vi "sync init shared memory.vi"(7 "permissions (0664)":T1={"owner"={"read"=TRUE, "write"=TRUE, "execute"=FALSE}, "group"={"read"=TRUE, "write"=TRUE, "execute"=FALSE}, "everyone"={"read"=TRUE, "write"=TRUE, "execute"=FALSE}}, 8 "error in (no error)":errorcluster, 11 "sync shm name":string) -> (0 "error out":errorcluster, 2 "pointer to shared memory":u64, 3 "shared memory out":T3)   [LabVIEW 2014, in "Shared Memory runtime.lvclass"]
uses:
  Shared Memory runtime.lvclass
  <vilib>/NI/NI Linux RT IPC/Shared Memory/Classes/Shared Memory/Public/Controls/reference.ctl
  <vilib>/NI/NI Linux RT IPC/Shared Memory/Classes/Shared Memory/Shared Memory.lvclass
  <vilib>/NI/NI Linux RT IPC/Shared Memory/Classes/Shared Memory/Public/Controls/permissions group.ctl
  <vilib>/NI/NI Linux RT IPC/Shared Memory/Classes/Shared Memory/Public/Controls/permissions.ctl
  <vilib>/NI/NI Linux RT IPC/Shared Memory/Classes/Shared Memory/Public/Controls/file mode.ctl
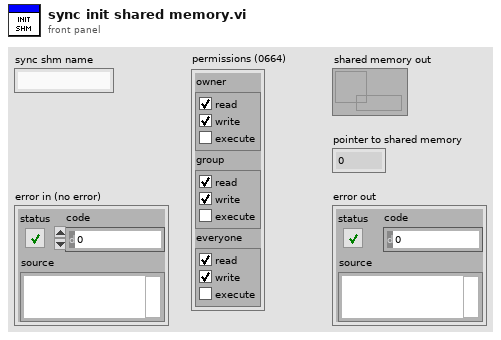
[diagram p1: front panel]
types:
  T1 = typedef "Shared Memory.lvlib/Shared Memory.lvclass/permissions group.ctl" = cluster{"owner":T2, "group":T2, "everyone":T2}
  T2 = typedef "Shared Memory.lvlib/Shared Memory.lvclass/permissions.ctl" = cluster{"read":bool, "write":bool, "execute":bool}
  T3 = typedef "Shared Memory.lvlib/Shared Memory.lvclass/reference.ctl" = refnum<data-value>
  T4 = typedef "Shared Memory.lvlib/Shared Memory.lvclass/file mode.ctl" = enum16{"open", "create/replace"}
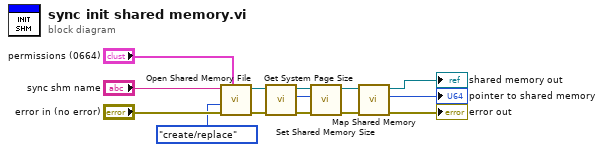
[diagram p0: block diagram]
diagram:
  n1 = call <vilib>:"Open Shared Memory File.vi"("permissions (0664)"="permissions (0664)", "error in (no error)"="error in (no error)", "file mode (open)"=file_mode."create/replace", "shared memory name"="sync shm name") -> ("error out"=w5:errorcluster, "shared memory out"=w6:T3)  [unwired: 6 in]
  n2 = call <vilib>:"Get System Page Size.vi"("error in (no error)"=w5, "shared memory in"=w6) -> ("error out"=w7:errorcluster, "page size (bytes)"=w9:u32, "shared memory out"=w8:T3)  [unwired: 7 in]
  n3 = call <vilib>:"Set Shared Memory Size.vi"("error in (no error)"=w7, "size (bytes)"=w9, "shared memory in"=w8) -> ("error out"=w11:errorcluster, "shared memory out"=w10:T3)  [unwired: 7 in]
  n4 = call <vilib>:"Map Shared Memory.vi"("error in (no error)"=w11, "shared memory in"=w10) -> ("error out"=→"error out":errorcluster, "pointer to shared memory"=→"pointer to shared memory":u64, "shared memory out"=→"shared memory out":T3)  [unwired: 7 in]
